vi "Configure Digital Input Noise.vi"(6 "EBNO Value (0 dB)":dbl, 7 "Carrier Bit Rate (1.000000E+0 bps)":dbl=1.0 format="%.6e", 8 "error in (no error)":errorcluster, 9 "Carrier to Noise Ratio (0.00000000E+0 dB)":dbl format="%.8e", 10 "Carrier to Noise Ratio Format (0: Carrier to Noise Ratio)":i32(ring) items=["Carrier to Noise Ratio", "Energy per Bit over Noise Power Density"], 11 "VISA resource name":refnum<visa-resource-name>) -> (0 "error out":errorcluster, 3 "VISA resource name out":refnum<visa-resource-name>)   [LabVIEW 2018, in "Agilent PSG MXG Series.lvlib"]
doc: "Configures the digital input noise settings.\n\n<b>Note:</b>\nIt is applicable for N5172B/82B with <b>Option 004</b> only."
uses:
  Agilent PSG MXG Series.lvlib
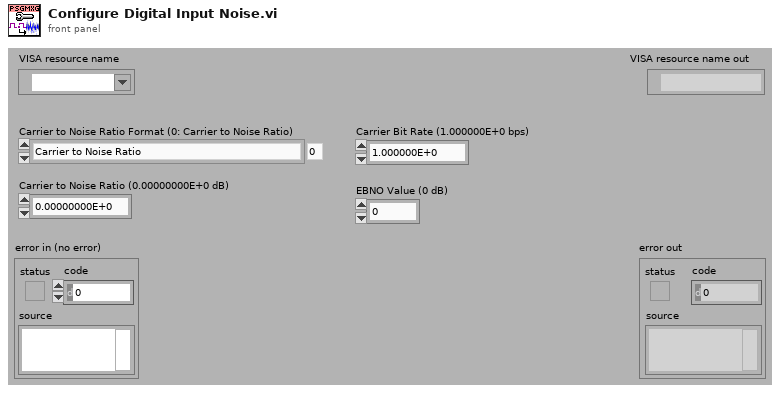
[diagram p1: front panel]
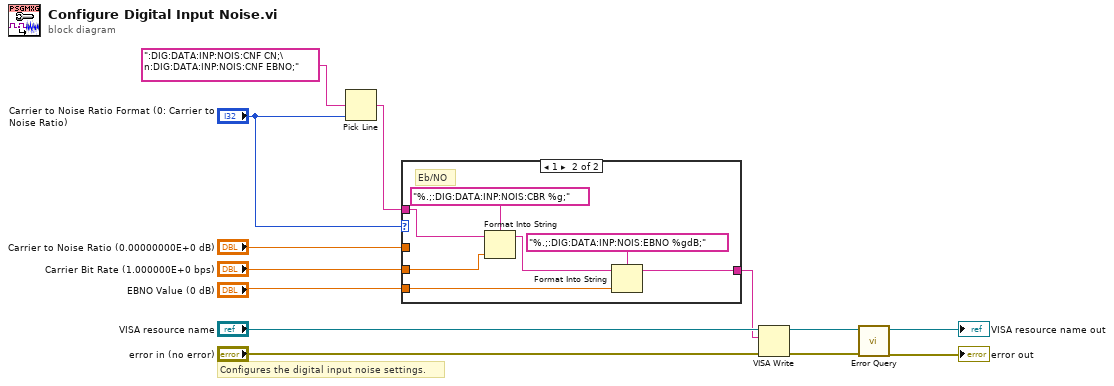
[diagram p0: block diagram]
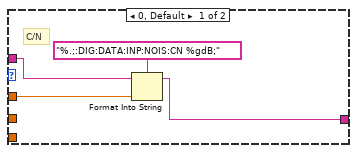
[diagram p2: hidden frame]
diagram:
  # "Configures the digital input noise settings."
  n1 = Pick Line(multi-line string=":DIG:DATA:INP:NOIS:CNF CN;\n:DIG:DATA:INP:NOIS:CNF EBNO;", line index="Carrier to Noise Ratio Format (0: Carrier to Noise Ratio)") -> (output string=w5:string)  [unwired: 1 in]
  n2 = case shown="1" "Carrier to Noise Ratio Format (0: Carrier to Noise Ratio)" {
    tunnel: w5 -> [w16 w22]
    tunnel: "Carrier to Noise Ratio (0.00000000E+0 dB)" -> [w15 _]
    tunnel: [w14 w18] -> w3
    tunnel: "Carrier Bit Rate (1.000000E+0 bps)" -> [_ w21]
    tunnel: "EBNO Value (0 dB)" -> [_ w19]
    frame 0, Default {
      # "C/N"
      n3 = Format Into String(format string="%.;:DIG:DATA:INP:NOIS:CN %gdB;", initial string=w16, w15) -> (resulting string=w14:string)  [unwired: 1 in, 1 out]
    }
    frame 1 {
      # "Eb/NO"
      n4 = Format Into String(format string="%.;:DIG:DATA:INP:NOIS:CBR %g;", initial string=w22, w21) -> (resulting string=w20:string)  [unwired: 1 in, 1 out]
      n5 = Format Into String(format string="%.;:DIG:DATA:INP:NOIS:EBNO %gdB;", initial string=w20, w19) -> (resulting string=w18:string)  [unwired: 1 in, 1 out]
    }
  }
  n6 = VISA Write(VISA resource name="VISA resource name", write buffer=w3, error in (no error)="error in (no error)") -> (VISA resource name out=w10:refnum<visa-resource-name>, error out=w9:errorcluster)  [unwired: 1 out]
  n7 = call "Error Query.vi"("error in (no error)"=w9, "VISA resource name"=w10) -> ("error out"=→"error out":errorcluster, "VISA resource name out"=→"VISA resource name out":refnum<visa-resource-name>)  [unwired: 6 in, 2 out]
